vi "XNET IP Stack Create.vi"(0 "config":string, 5 "stack name":string, 11 "error in":errorcluster) -> (4 "stack out":refnum<k21>, 15 "error out":errorcluster)   [LabVIEW 2018]
doc: "Creates an XNET IP stack to use for TCP and/or UDP communication."
uses:
  nixlvapi.dll
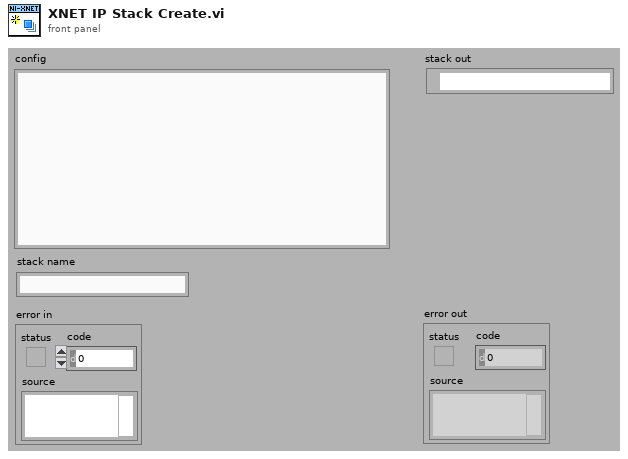
[diagram p1: front panel]
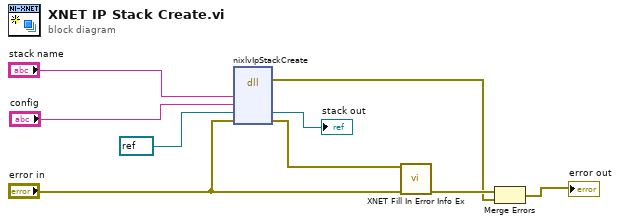
[diagram p0: block diagram]
diagram:
  n1 = dll-call lib="nixlvapi.*" fn="nixlvIpStackCreate" label="Call Library"("stackName"="stack name", "config"="config", "stack out"=refnum<k21> refnum ("XNET Frame"), "errorInOut"="error in") -> (error out=w2:errorcluster, "stack out"=→"stack out":refnum<k21>, "errorInOut"=w8:errorcluster)  [unwired: 3 in, 4 out]
  n2 = call "XNET Fill In Error Info Ex.vi"("error xnet"=w8, "error in"="error in") -> ("error out"=w3:errorcluster)  [unwired: 13 in]
  n3 = Merge Errors(w3, w2) -> (→"error out":errorcluster)
